vi "ARRAY OF CLUSTERS.vi"() -> ()   [LabVIEW 2018]
panel:
  out "Array 2":T1(array[cluster])
  in  "Array":T1(array[cluster])
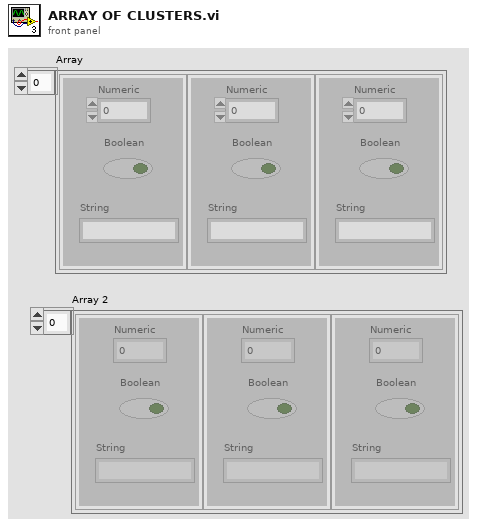
[diagram p1: front panel]
types:
  T1 = cluster{"Numeric":dbl, "Boolean":bool, "String":string}[]
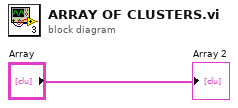
[diagram p0: block diagram]
diagram:
  "Array 2" <- "Array"
